vi "Write dEL_ArcsPS.vi"(8 "error in (no error)":errorcluster, 10 "dEL_ArcsPS":dbl[unit] min=-4.84813681109536e-05 max=4.84813681109536e-05, 11 "DifftrackAzEl in":refnum<class "DifftrackAzEl.lvclass">) -> (0 "error out":errorcluster, 3 "DifftrackAzEl out":refnum<class "DifftrackAzEl.lvclass">)   [LabVIEW 2022 SP3, in "TCSDataDefinitions.lvlib" / "TCSCommand.lvlib" / "TargetConfiguration.lvlib" / "Target.lvlib" / "DifftrackAzEl.lvclass"]
uses:
  DifftrackAzEl.lvclass
  DifftrackAzEl.lvclass/DifftrackAzEl.ctl
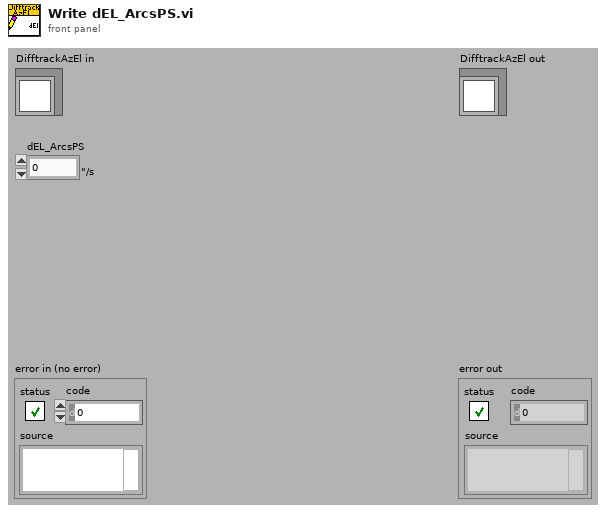
[diagram p1: front panel]
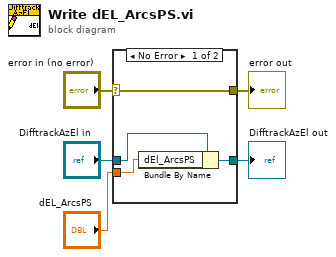
[diagram p0: block diagram]
diagram:
  n1 = case shown="No Error" "error in (no error)" {
    selector: "error in (no error)" -> [w9 w10]
    tunnel: [w9 w10] -> w4
    tunnel: [w7 w11] -> w2
    tunnel: "DifftrackAzEl in" -> [w8 w11]
    tunnel: "dEL_ArcsPS" -> [w6 _]
    frame No Error {
      n2 = Bundle By Name(cluster=w8, "dEl_ArcsPS"=w6) -> (w7:refnum<class "DifftrackAzEl.lvclass">)
    }
    frame Error {
    }
  }
  "error out" <- w4
  "DifftrackAzEl out" <- w2
